vi "Case_structure_for_months.vi"() -> ()   [LabVIEW 2019]
panel:
  in  "Month":u8
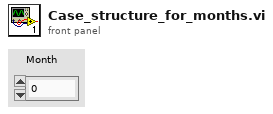
[diagram p1: front panel]
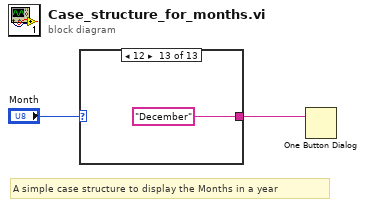
[diagram p0: block diagram]
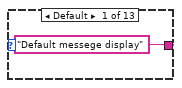
[diagram p2: hidden frame]
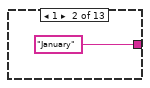
[diagram p3: hidden frame]
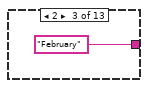
[diagram p4: hidden frame]
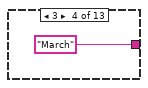
[diagram p5: hidden frame]
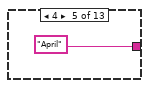
[diagram p6: hidden frame]
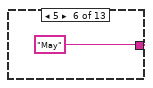
[diagram p7: hidden frame]
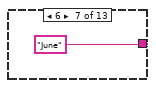
[diagram p8: hidden frame]
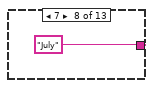
[diagram p9: hidden frame]
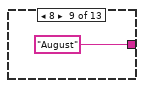
[diagram p10: hidden frame]
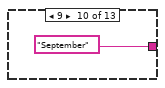
[diagram p11: hidden frame]
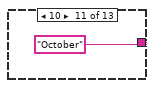
[diagram p12: hidden frame]
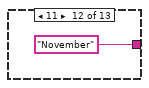
[diagram p13: hidden frame]
diagram:
  # "A simple case structure to display the Months in a year"
  n1 = case shown="12" "Month" {
    tunnel: ["Default messege display" "January" "February" "March" "April" "May" "June" "July" "August" "September" "October" "November" "December"] -> w2
    frame Default {
    }
    frame 1 {
    }
    frame 2 {
    }
    frame 3 {
    }
    frame 4 {
    }
    frame 5 {
    }
    frame 6 {
    }
    frame 7 {
    }
    frame 8 {
    }
    frame 9 {
    }
    frame 10 {
    }
    frame 11 {
    }
    frame 12 {
    }
  }
  n2 = One Button Dialog(message=w2) -> ()  [unwired: 1 in, 1 out]
